vi "Changing Panels Launcher.vi"   [LabVIEW 2017, in "2. Basic Panel Actors.lvlib"]
doc: "Launches the Chaning Panel Example.\n----\nCopyright: MGI 2017\nAuthor: Derek Trepanier"
uses:
  2. Basic Panel Actors.lvlib
  Changing Panels/Changing Panels.lvclass
  D:/software/LabView_PanelManager/panel-actors/Source/Panel Actor/Panel Actor.lvclass
  panel-manager/Source/Window Position/Reference Position/Alignment.ctl
  panel-manager/Source/Window Position/Reference Position/Horizontal Alignment.ctl
  panel-manager/Source/Window Position/Reference Position/Vertical Alignment.ctl
  panel-manager/Source/Window Position/Reference Position/Offset/Absolute Offset/No Offset.vi
  panel-manager/Source/Window Position/Reference Position/Offset/Absolute Offset/Absolute Offset.lvclass
  D:/software/LabView_PanelManager/panel-manager/Source/Window Position/Reference Position/Offset/Offset.lvclass
  panel-manager/Source/Window Position/Reference Position/Ref Display/Ref Display.lvclass
  D:/software/LabView_PanelManager/panel-manager/Source/Window Position/Window Position.lvclass
  panel-manager/Source/Window Position/Reference Position/Ref Display/Ref Display.vi
  panel-actors/Source/Launch Root Panel Window.vi
  panel-manager/Source/MGI-Panel Manager.lvlib
  panel-manager/Source/Window Position/Reference Position/Reference Position.lvclass
  panel-actors/Source/MGI-Panel Actor.lvlib
  D:/software/LabView_PanelManager/panel-manager/Source/Window Position/Reference Position/Reference Position.lvclass
  C:/Program Files (x86)/National Instruments/LabVIEW 2017/vi.lib/ActorFramework/Actor/Actor.lvclass
panel:
  # "Run this VI to launch the Changing Panel example."
types:
  T1 = typedef "MGI-Panel Manager.lvlib/Reference Position.lvclass/Alignment.ctl" = cluster{"Horizontal":T2, "Vertical":T3}
  T2 = typedef "MGI-Panel Manager.lvlib/Reference Position.lvclass/Horizontal Alignment.ctl" = enum16{"Left", "Center", "Right"}
  T3 = typedef "MGI-Panel Manager.lvlib/Reference Position.lvclass/Vertical Alignment.ctl" = enum16{"Top", "Center", "Bottom"}
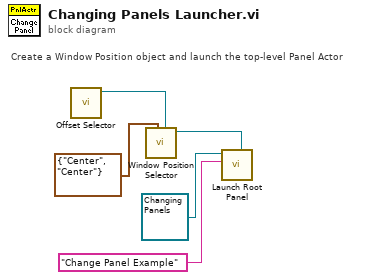
[diagram p0: block diagram]
diagram:
  # "Create a Window Position object and launch the top-level Panel Actor"
  n1 = call-poly "Offset Selector.vi"() -> ("Absolute Offset Out"=w3:refnum<class "Absolute Offset.lvclass">)  [unwired: 10 in, 1 out]
  n2 = call-poly "Window Position Selector.vi"("Offset"=w3, "Alignment"=T1 {"Horizontal"=enum."Center", "Vertical"=enum."Center"}) -> ("Ref Display out"=w4:refnum<class "Ref Display.lvclass">)  [unwired: 8 in, 1 out]
  n3 = call-poly "Launch Root Panel.vi"("Window Position (Maximize First Call)"=w4, "Title"="Change Panel Example", "Panel Actor in"=refnum<class "Changing Panels.lvclass"> refnum ("2. Basic Panel Actors.lvlib:Changing Panels.lvclass")) -> ()  [unwired: 7 in, 2 out]
